vi "read_raw.vi"() -> ()   [LabVIEW 2015]
uses:
  <vilib>/FPGAPlugInAG/USB-7855R OEM/niLvFpga_Open_USB-7855R OEM.vi
  <vilib>/rvi/interface/common/dynamic/niFpgaDynamicAddResources.vi
  <vilib>/Utility/error.llb/Error Cluster From Error Code.vi
  <vilib>/rvi/errors/niLvFpgaAdjustHostInterfaceError.vi
  <vilib>/FPGAPlugInAG/Dynamic/niLvFpga_Close_Dynamic.vi
  <vilib>/rvi/interface/nirviOpenFPGA/nirviOpenFPGA.xnode
  FPGA Bitfiles/hydrophones_FPGATarget_tdoa_yTCOovIDrm4.lvbitx
  tdoa.vi
  <vilib>/rvi/interface/nirviMethod/nirviMethod.xnode
  <vilib>/rvi/interface/nirviCloseFPGA/nirviCloseFPGA.xnode
  <vilib>/FPGAPlugInAG/Dynamic/niLvFpga_ReadFifo_Dynamic.vi
  <vilib>/rvi/errors/niLvFpgaMergeErrorWithErrorCode.vi
panel:
  out "signal4":waveform(i16)(graph)
  out "signal3":waveform(i16)(graph)
  out "signal2":waveform(i16)(graph)
  out "signal1":waveform(i16)(graph)
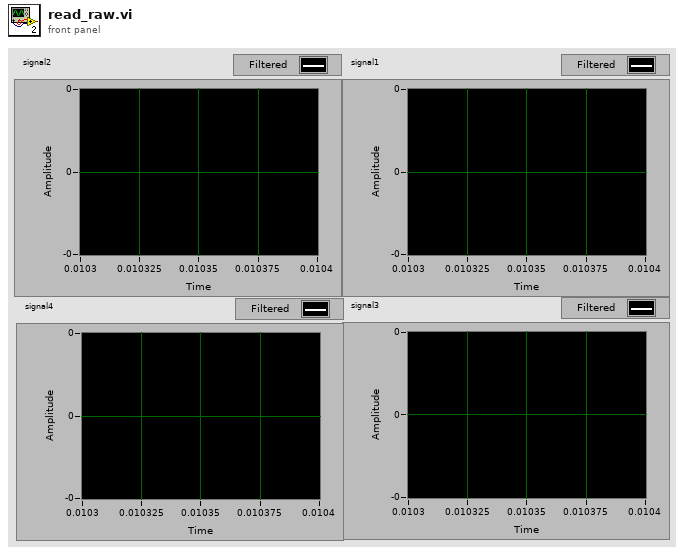
[diagram p1: front panel]
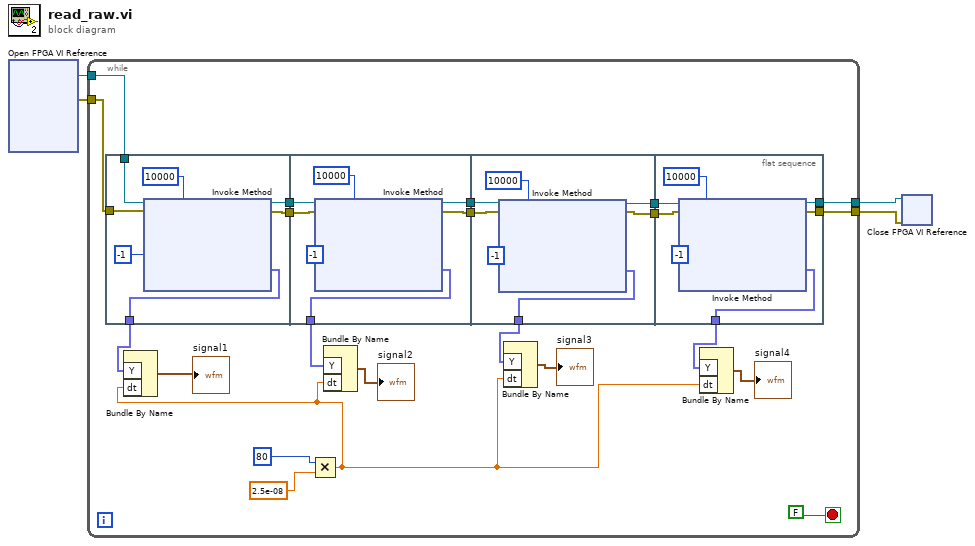
[diagram p0: block diagram]
diagram:
  n1 = xnode "Open FPGA VI Reference"() -> ("FPGA VI Reference Out"=w4:refnum<k20>, "error out"=w3:errorcluster)  [unwired: 2 in]
  n2 = while {
    tunnel: w4 -> [w25]
    tunnel: w3 -> [w24]
    tunnel: [w17] -> w2
    tunnel: [w16] -> w1
    stop <- FALSE stop-if-true
    n3 = flat-sequence {
      tunnel: w25 -> [w33]
      tunnel: w24 -> [w32]
      tunnel: [w29] -> w15
      tunnel: [w28] -> w23
      tunnel: [w27] -> w22
      tunnel: w23 -> [w40]
      tunnel: w22 -> [w39]
      tunnel: [w38] -> w13
      tunnel: [w37] -> w21
      tunnel: [w36] -> w20
      tunnel: w21 -> [w47]
      tunnel: w20 -> [w46]
      tunnel: [w45] -> w11
      tunnel: [w42] -> w19
      tunnel: [w41] -> w18
      tunnel: w19 -> [w54]
      tunnel: w18 -> [w53]
      tunnel: [w50] -> w9
      tunnel: [w49] -> w17
      tunnel: [w48] -> w16
      frame #0 {
        n4 = xnode "Invoke Method"("FPGA VI Reference In"=w33, "error in"=w32, "Number of Elements"=u32 10000, "Timeout (ms)"=-1) -> ("FPGA VI Reference Out"=w28:refnum<k20>, "error out"=w27:errorcluster, "Data"=w29:fxp<+/-,16,16>[])  [unwired: 1 out]
      }
      frame #1 {
        n5 = xnode "Invoke Method"("FPGA VI Reference In"=w40, "error in"=w39, "Number of Elements"=u32 10000, "Timeout (ms)"=-1) -> ("FPGA VI Reference Out"=w37:refnum<k20>, "error out"=w36:errorcluster, "Data"=w38:fxp<+/-,16,16>[])  [unwired: 1 out]
      }
      frame #2 {
        n6 = xnode "Invoke Method"("FPGA VI Reference In"=w47, "error in"=w46, "Number of Elements"=u32 10000, "Timeout (ms)"=-1) -> ("FPGA VI Reference Out"=w42:refnum<k20>, "error out"=w41:errorcluster, "Data"=w45:fxp<+/-,16,16>[])  [unwired: 1 out]
      }
      frame #3 {
        n7 = xnode "Invoke Method"("FPGA VI Reference In"=w54, "error in"=w53, "Number of Elements"=u32 10000, "Timeout (ms)"=-1) -> ("FPGA VI Reference Out"=w48:refnum<k20>, "error out"=w49:errorcluster, "Data"=w50:fxp<+/-,16,16>[])  [unwired: 1 out]
      }
    }
    n8 = Multiply(x=80, y=2.5e-08) -> (x*y=w5:dbl)
    n9 = Bundle By Name("Y"=w15, "dt"=w5) -> (→"signal1":waveform(i16))  [unwired: 1 in]
    n10 = Bundle By Name("Y"=w13, "dt"=w5) -> (→"signal2":waveform(i16))  [unwired: 1 in]
    n11 = Bundle By Name("Y"=w11, "dt"=w5) -> (→"signal3":waveform(i16))  [unwired: 1 in]
    n12 = Bundle By Name("Y"=w9, "dt"=w5) -> (→"signal4":waveform(i16))  [unwired: 1 in]
  }
  n13 = xnode "Close FPGA VI Reference"("FPGA VI Reference In"=w1, "error in"=w2) -> ()  [unwired: 1 out]
